vi "Main.vi"() -> ()   [LabVIEW 2015]
doc: "The myRIO Project template acquires acceleration data from the onboard accelerometer and displays the changes of acceleration values in a waveform chart."
uses:
  <vilib>/myRIO/Instrument Drivers/Utilities/Utilities.lvlib
  <vilib>/myRIO/Express VI/Onboard Devices/Accelerometer/Accelerometer Express VI.xnode
  <vilib>/myRIO/Instrument Drivers/Onboard Devices/Accelerometer/vis/Read.vi
  <vilib>/myRIO/Instrument Drivers/Onboard Devices/Accelerometer/Accelerometer.lvlib
  <vilib>/myRIO/Common/Instrument Driver Framework/myRIO v1.0/Accelerometer/typedefs/Accelerometer Channels Enum.ctl
  <vilib>/myRIO/Common/Instrument Driver Framework/myRIO v1.0/Accelerometer/typedefs/Accelerometer Channels List.ctl
  <vilib>/myRIO/Common/Instrument Driver Framework/Utilities/typedefs/Generic FPGA Reference.ctl
  <vilib>/myRIO/Common/Instrument Driver Framework/Utilities/typedefs/myRIO v1.0 Reference.ctl
  <vilib>/myRIO/Common/Instrument Driver Framework/Utilities/typedefs/Hardware Version Enum.ctl
  <vilib>/myRIO/Common/Instrument Driver Framework/Utilities/typedefs/myRIO Generic Hardware Reference.ctl
  <vilib>/myRIO/Instrument Drivers/Onboard Devices/Accelerometer/typedefs/Accelerometer Reference.ctl
  <vilib>/myRIO/Instrument Drivers/Onboard Devices/Accelerometer/vis/myRIO Accelerometer Open.xnode
  <vilib>/myRIO/Common/Instrument Driver Framework/Utilities/vis/Is FPGA Ref Available.vi
  <vilib>/myRIO/Common/Instrument Driver Framework/myRIO v1.0/Accelerometer/vis/myRIO v1.1 Open Accelerometer.vi
  <vilib>/userdefined/High Color/nirio_resource_hc.ctl
  <vilib>/vision/NI_Vision_Development_Module.lvlib
  <vilib>/vision/driver/NI_Vision_Acquisition_Software.lvlib
  <vilib>/userdefined/High Color/IMAQdx.ctl
  <vilib>/vision/Pattern Matching.llb/IMAQ GM Match Report.ctl
  <vilib>/vision/Pattern Matching.llb/IMAQ Match Range Setting.ctl
  <vilib>/vision/Pattern Matching.llb/IMAQ Curve Parameters.ctl
panel:
  in  "BCG Values":T1={"Brightness"=128.0, "Contrast"=45.0, "Gamma"=1.0} {"Brightness" min=0 max=255 step=1 format="%.2f"; "Contrast" min=1 max=89 step=1 format="%.2f"; "Gamma" min=0.1 max=10 step=0.01 format="%.2f"}
  in  "Curve Parameters":T2={"Extraction Mode"=0, "Edge Threshold"=75, "Edge Filter Size"=1, "Min Length"=25, "Row Search Step Size"=15, "Col Search Step Size"=15, "Max Endpoint Gap"=10, "Closed"=FALSE, "Subpixel"=FALSE} {"Extraction Mode" items=["Normal", "Uniform Regions"]; "Edge Filter Size" items=["Fine", "Normal", "Contour Tracing"]; "Max Endpoint Gap" min=0; "Col Search Step Size" min=1 max=255 step=1; "Row Search Step Size" min=1 max=255 step=1; "Min Length" min=0; "Edge Threshold" min=1 max=350 step=1}
  in  "Advanced Geometric Learn Options 2":T3(array[cluster]) {"Item Value" format="%.2f"; "Setup Data Item" items=["Curve Extraction Mode", "Curve Edge Threshold", "Curve Edge Filter Size", "Min Curve Length", "Curve Row Search Step Size", "Curve Col Search Step Size", "Curve Max Endpoint Gap", "Extract Closed Curves", "Enable Supixel Curve Extraction", "Minimum Scale Factor (%)", "Maximum Scale Factor (%)", "Minimum Angle Value", "Maximum Angle Value", "Image Sampling Factor", "Use All Curves"]}
  in  "Angle Offset":sgl min=-360 max=360 format="%.2f"
  in  "Origin Offset":cluster{"X":sgl, "Y":sgl} {"Y" format="%.2f"; "X" format="%.2f"}
  in  "Range Settings":T4[](array[typedef]) {"Max" format="%.2f"; "Min" format="%.2f"; "Match Constraints" items=["Rotation Angle (degrees)", "Scale Factor (%)", "Occlusion (%)"]}
  out "Number of Matches":i32
  out "Matches (pixel)":T5[](array[typedef]) {"Correlation Score" format="%.2f"; "Target Template Curve Score" format="%.2f"; "Template Target Curve Score" format="%.2f"; "Bounding Box"."y" format="%.2f"; "Bounding Box"."x" format="%.2f"; "Position"."y" format="%.2f"; "Position"."x" format="%.2f"; "Score" format="%.2f"; "Scale" format="%.2f"; "Angle" format="%.2f"; "Occlusion %" format="%.2f"}
  out "Acceleration":T6(graph)
  out "error out":errorcluster
  in  "Stop":bool
  # "Overview: The myRIO Project template acquires acceleration data from the onboard accelerometer and displays the changes of acceleration values in a waveform chart.\nInstructions:\n1. Check the myRIO target IP address in the project and make sure the target IP address is correct. \n2. Run this VI."
  # "Range"
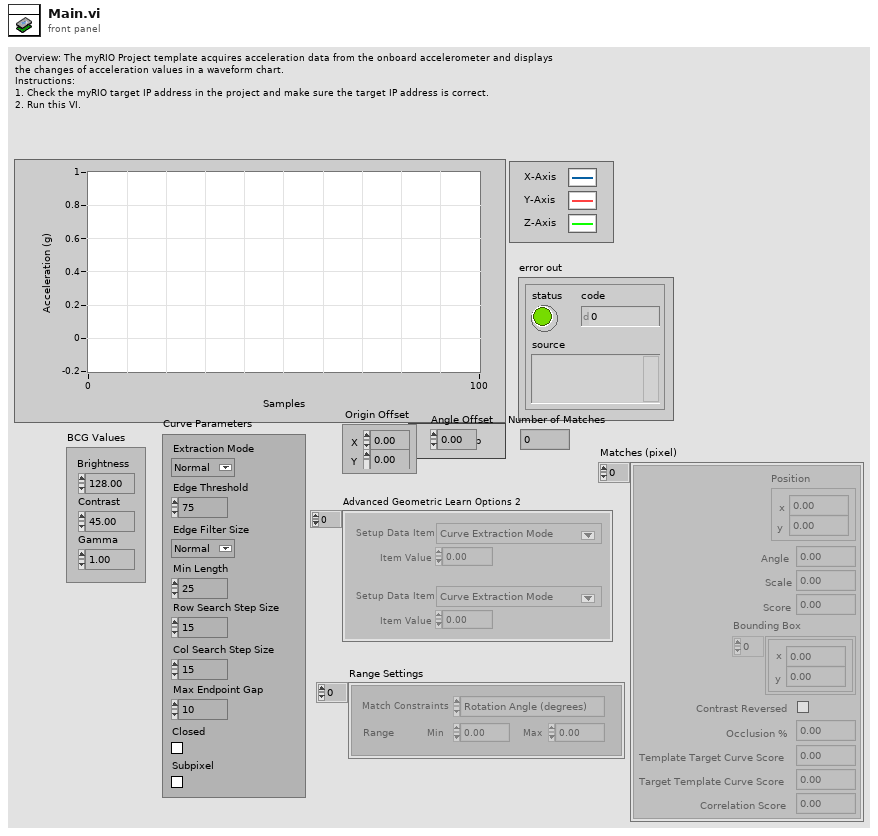
[diagram p1: front panel]
types:
  T1 = cluster{"Brightness":sgl, "Contrast":sgl, "Gamma":sgl}
  T2 = typedef "IMAQ Curve Parameters.ctl" = cluster{"Extraction Mode":u32, "Edge Threshold":i32, "Edge Filter Size":u32, "Min Length":i32, "Row Search Step Size":i32, "Col Search Step Size":i32, "Max Endpoint Gap":i32, "Closed":bool, "Subpixel":bool}
  T3 = cluster{"Setup Data Item":u16, "Item Value":dbl}[]
  T4 = typedef "IMAQ Match Range Setting.ctl" = cluster{"Match Constraints":u32, "Min":dbl, "Max":dbl}
  T5 = typedef "IMAQ GM Match Report.ctl" = cluster{"Position":cluster{"x":sgl, "y":sgl}, "Angle":sgl, "Scale":sgl, "Score":sgl, "Bounding Box":cluster{"x":sgl, "y":sgl}[], "Contrast Reversed":bool, "Occlusion %":sgl, "Template Target Curve Score":sgl, "Target Template Curve Score":sgl, "Correlation Score":sgl}
  T6 = cluster{"X-Axis":dbl, "Y-Axis":dbl, "Z-Axis":dbl}
  T7 = typedef "IMAQdx.ctl" = refnum<k21>
  T8 = typedef "Accelerometer.lvlib/Accelerometer Reference.ctl" = cluster{"myRIO Reference":T9, "Accelerometer Channels List":T13, "LSB Weight":dbl}
  T9 = typedef "myRIO Generic Hardware Reference.ctl" = cluster{"myRIO Model":T10, "myRIO Hardware Reference":T11}
  T10 = typedef "Hardware Version Enum.ctl" = enum16{"Unknown", "myRIO-1900", "myRIO-1950", "roboRIO"}
  T11 = typedef "myRIO v1.0 Reference.ctl" = cluster{"Generic FPGA Reference":T12, "Allow multiple opens":bool}
  T12 = typedef "Generic FPGA Reference.ctl" = refnum<k20>
  T13 = typedef "Accelerometer Channels List.ctl" = T14[]
  T14 = typedef "Accelerometer Channels Enum.ctl" = enum16{"Not Connected", "X-Axis", "Y-Axis", "Z-Axis"}
  T15 = typedef "nirio_resource_hc.ctl" = tag
  T16 = typedef "Image Type" = u32
  T17 = typedef "IMAQ Image.ctl" = refnum<image>
  T18 = typedef "imagedata.ctl" = cluster{"image type":i32, "image depth":i32, "image":u8[], "mask":u8[], "colors":u32[], "Rectangle":cluster{"left":i16, "top":i16, "right":i16, "bottom":i16}}
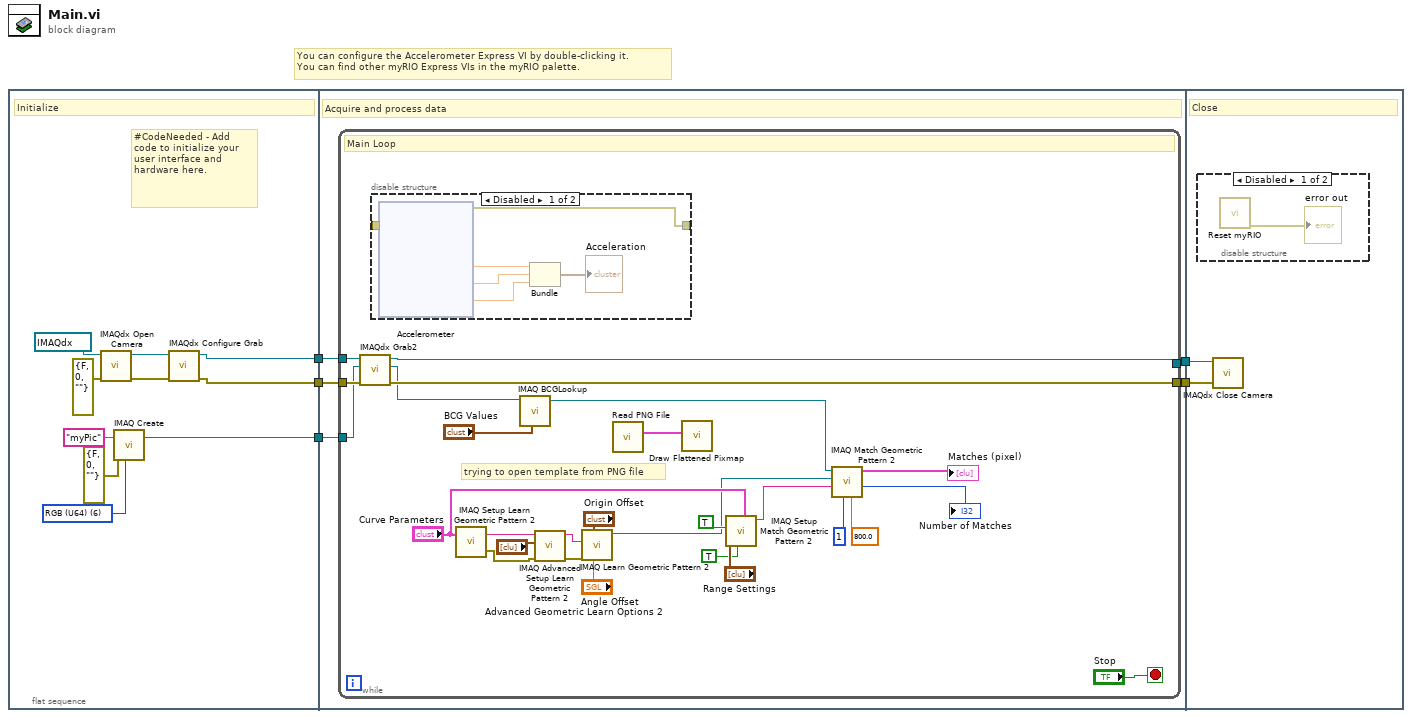
[diagram p0: block diagram]
diagram:
  # "You can configure the Accelerometer Express VI by double-clicking it.\nYou can find other myRIO Express VIs in the myRIO palette."
  n1 = flat-sequence {
    tunnel: [w8] -> w5
    tunnel: [w7] -> w4
    tunnel: [w6] -> w3
    tunnel: w5 -> [w20]
    tunnel: w4 -> [w19]
    tunnel: w3 -> [w18]
    tunnel: [w17] -> w2
    tunnel: [w16] -> w1
    tunnel: w2 -> [w94]
    tunnel: w1 -> [w93]
    frame #0 {
      w13 = T16 6 items=["Grayscale (U8)", "Grayscale (I16)", "Grayscale (SGL)", "Complex (CSG)", "RGB (U32)", "HSL (U32)", "RGB (U64)", "Grayscale (U16)"] ("Image Type")
      # "#CodeNeeded - Add code to initialize your user interface and hardware here."
      # "Initialize"
      n2 = call <vilib>:"IMAQdx Open Camera.vi"("error in"=errorcluster {"status"=FALSE, "code"=0, "source"=""}, "Session In"=T7 "cam0") -> ("error out"=w14:errorcluster, "Session Out"=w15:T7)  [unwired: 8 in]
      n3 = call "IMAQ Create"("Image Name"="myPic", "Image Type"=w13, "error in (no error)"=errorcluster {"status"=FALSE, "code"=0, "source"=""}) -> ("New Image"=w6:T17)  [unwired: 2 in, 1 out]
      n4 = call <vilib>:"IMAQdx Configure Grab.vi"("error in"=w14, "Session In"=w15) -> ("error out"=w7:errorcluster, "Session Out"=w8:T7)  [unwired: 8 in]
    }
    frame #1 {
      # "Acquire and process data"
      n5 = while {
        tunnel: w20 -> [w29]
        tunnel: w19 -> [w28]
        tunnel: w18 -> [w27]
        tunnel: [w26] -> w17
        tunnel: [w25] -> w16
        stop <- "Stop" stop-if-true
        # "trying to open template from PNG file"
        # "Main Loop"
        n6 = call <vilib>:"IMAQdx Grab2.vi"("error in"=w28, "Image In"=w27, "Session In"=w29) -> ("error out"=w25:errorcluster, "Image Out"=w24:T17, "Session Out"=w26:T7)  [unwired: 5 in, 1 out]
        n7 = disable-structure shown="Disabled" {
          disable-tunnel: _ -> [w52 _]
          disable-tunnel: [w51 _] -> _
          frame Disabled {
            n8 = xnode "Accelerometer"("error in (no error)"=w52) -> ("X-Axis"=w50:dbl, "Y-Axis"=w49:dbl, "Z-Axis"=w48:dbl, "error out"=w51:errorcluster)
            n9 = Bundle("X-Axis"=w50, "Y-Axis"=w49, "Z-Axis"=w48) -> (→"Acceleration":T6)  [unwired: 1 in]
          }
          frame Enabled {
          }
        }
        n10 = call "IMAQ Setup Learn Geometric Pattern 2"("Curve Parameters"="Curve Parameters") -> ("error out"=w45:errorcluster, "Learn Geometric Pattern 2 Setup Data"=w47:string)  [unwired: 1 in]
        n11 = call "IMAQ BCGLookup"("Image Src"=w24, "BCG Values"="BCG Values") -> ("Image Dst Out"=w22:T17)  [unwired: 5 in, 1 out]
        n12 = call "IMAQ Advanced Setup Learn Geometric Pattern 2"("Learn Geometric Pattern 2 Setup Data In"=w47, "Advanced Geometric Learn Options 2"="Advanced Geometric Learn Options 2", "error in (no error)"=w45) -> ("Learn Geometric Pattern 2 Setup Data Out"=w46:string, "error out"=w44:errorcluster)  [unwired: 6 in]
        n13 = call "IMAQ Learn Geometric Pattern 2"("Angle Offset"="Angle Offset", "Origin Offset"="Origin Offset", "error in (no error)"=w44, "Learn Geometric Pattern 2 Setup Data"=w46) -> ("Template Image Out"=w35:T17)  [unwired: 6 in, 1 out]
        n14 = call <vilib>:"Read PNG File.vi"() -> ("image data"=w21:T18)  [unwired: 9 in, 2 out]
        n15 = call <vilib>:"Draw Flattened Pixmap.vi"("image data"=w21) -> ()  [unwired: 8 in, 1 out]
        n16 = call "IMAQ Setup Match Geometric Pattern 2"("Use Learn Curve Parameters"=TRUE, "Curve Parameters"="Curve Parameters", "Range Settings"="Range Settings", "Subpixel Accuracy"=TRUE) -> ("Match Geometric Pattern 2 Setup Data"=w36:string)  [unwired: 6 in, 1 out]
        n17 = call "IMAQ Match Geometric Pattern 2"("Minimum Match Score"=sgl 800.0, "Number of Matches Requested"=1, "Match Geometric Pattern 2 Setup Data"=w36, "Template Image"=w35, "Image"=w22) -> ("Number of Matches"=→"Number of Matches":i32, "Matches (pixel)"=→"Matches (pixel)":T5[])  [unwired: 3 in, 2 out]
      }
    }
    frame #2 {
      # "Close"
      n18 = disable-structure shown="Disabled" {
        frame Disabled {
          n19 = call <vilib>:"Reset myRIO.vi"() -> ("error out"=→"error out":errorcluster)  [unwired: 11 in]
        }
        frame Enabled {
        }
      }
      n20 = call <vilib>:"IMAQdx Close Camera.vi"("error in"=w93, "Session In"=w94) -> ()  [unwired: 9 in, 1 out]
    }
  }
